vi "Write to HW.vi"(11 "Plugin Framework in":refnum<class "Plugin Framework.lvclass">) -> (0 "error out":errorcluster, 3 "Plugin Framework out":refnum<class "Plugin Framework.lvclass">)   [LabVIEW 2024, in "Plugin Framework.lvclass"]
uses:
  Plugin Framework.lvclass
  Plugin Framework.lvclass/Plugin Framework.ctl
  Plugin/Plugin.lvclass
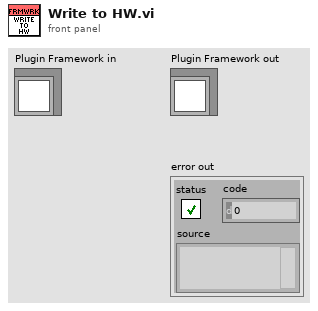
[diagram p1: front panel]
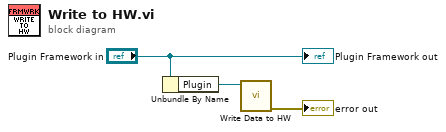
[diagram p0: block diagram]
diagram:
  n1 = Unbundle By Name("Plugin Framework in") -> ("Plugin"=w1:refnum<class "Plugin.lvclass">)
  n2 = call "Write Data to HW.vi"("Plugin in"=w1) -> ("error out"=→"error out":errorcluster)  [unwired: 9 in, 1 out]
  "Plugin Framework out" <- "Plugin Framework in"
